vi "Update Index Selector.vi"(8 "error in (no error)":errorcluster, 10 "Index selector":i32=-1, 11 "Monkey in":refnum<class "Monkey.lvclass">) -> (0 "error out":errorcluster, 3 "Monkey out":refnum<class "Monkey.lvclass">)   [LabVIEW 2020, in "Monkey.lvlib" / "Monkey.lvclass"]
uses:
  Monkey.lvclass
  Monkey.lvclass/Monkey.ctl
  Run Utilities/Run Block/Run Block.lvclass
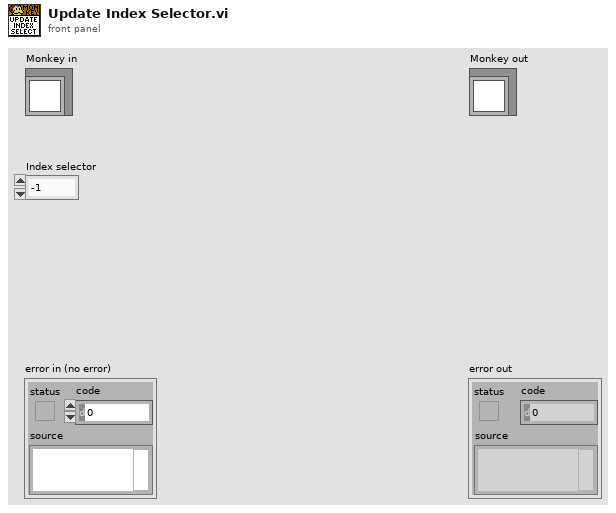
[diagram p1: front panel]
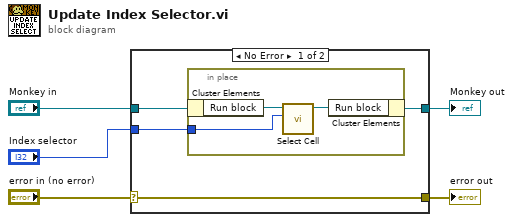
[diagram p0: block diagram]
diagram:
  n1 = case shown="No Error" "error in (no error)" {
    selector: "error in (no error)" -> [w7 w14]
    tunnel: [w7 w14] -> w4
    tunnel: [w8 w13] -> w2
    tunnel: "Monkey in" -> [w9 w13]
    tunnel: "Index selector" -> [w6 _]
    frame No Error {
      n2 = in-place {
        in-place-border: w6 -> [w10]
        n3 = in-place-cluster #1(w9) -> ("Run block"=w12:refnum<class "Run Block.lvclass">)
        n4 = call-dynamic "Select Cell.vi"("Index selector"=w10, "Run Block in"=w12) -> ("Run Block out"=w11:refnum<class "Run Block.lvclass">)  [unwired: 8 in, 1 out]
        n5 = in-place-cluster #1("Run block"=w11) -> (w8:refnum<class "Monkey.lvclass">)
      }
    }
    frame Error {
    }
  }
  "error out" <- w4
  "Monkey out" <- w2
